vi "Get Referenced NI-XNET Port Item IDs.vi"(8 "Error In":errorcluster, 10 "CD Port Item Ref In":T1 format="%.0x", 11 "Device Item Ref in in":T1 format="%.0x") -> (0 "Error Out":errorcluster, 1 "NI-XNET Port Item Ref Out":T1 format="%.0x", 3 "Device Item Ref out":T1 format="%.0x", 4 "Found?":bool)   [LabVIEW 2017, in "NI-XNET Monitor System Explorer.lvlib"]
uses:
  NI-XNET Monitor System Explorer.lvlib
  <vilib>/NI Veristand/Custom Device API/Custom Device Item Ref.ctl
  Shared/Constants.vi
  <vilib>/NI Veristand/Custom Device API/Get Item Property (String).vi
  <vilib>/NI Veristand/Custom Device API/Custom Device API.lvlib
  Shared/NI-XNET Monitor Shared.lvlib
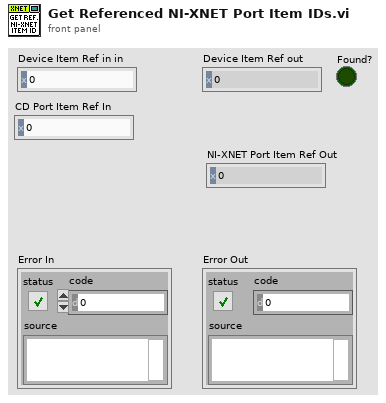
[diagram p1: front panel]
types:
  T1 = typedef "Custom Device API.lvlib/Custom Device Item Ref.ctl" = u64
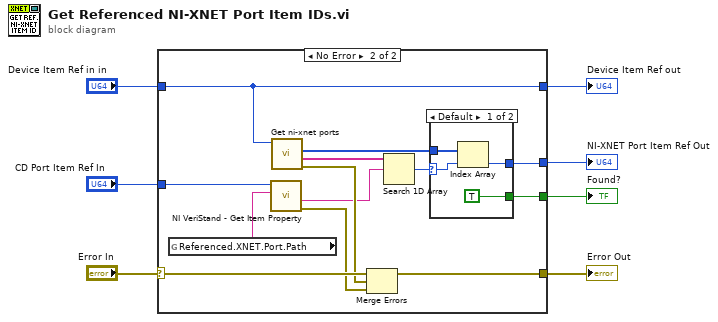
[diagram p0: block diagram]
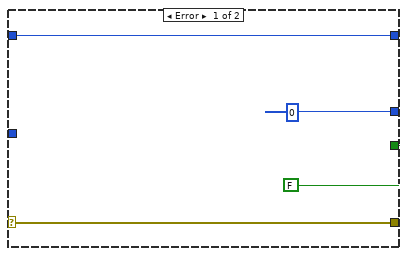
[diagram p2: hidden frame]
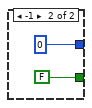
[diagram p3: hidden frame]
diagram:
  n1 = case shown="No Error" "Error In" {
    selector: "Error In" -> [w9 w24]
    tunnel: [w9 w23] -> w5
    tunnel: "Device Item Ref in in" -> [w11 w21]
    tunnel: [w11 w21] -> w7
    tunnel: "CD Port Item Ref In" -> [_ w17]
    tunnel: [T1 0 ("CD Port Item Ref In") w14] -> w2
    tunnel: [FALSE w13] -> w1
    frame Error {
    }
    frame No Error {
      n2 = global read "Constants.vi" "Referenced.XNET.Port.Path"() -> (w18:string)
      n3 = call-poly <vilib>:"NI VeriStand - Get Item Property.vi"("Property Name"=w18, "Item Ref in"=w17) -> ("error out"=w16:errorcluster, "Value"=w15:string)  [unwired: 6 in, 2 out]
      n4 = call "Get ni-xnet ports.vi"("Device Item Ref in"=w21) -> ("Error Out"=w22:errorcluster, "NI-XNET Port Item Paths"=w20:string[], "NI-XNET Port Refs"=w19:T1[])  [unwired: 7 in, 1 out]
      n5 = Merge Errors(w24, w22, w16) -> (w23:errorcluster)
      n6 = Search 1D Array(1D array=w20, element=w15) -> (index of element=w12:i32)  [unwired: 1 in]
      n7 = case shown="Default" w12 {
        selector: w12 -> [w27 _]
        tunnel: w19 -> [w28 _]
        tunnel: [w26 T1 0 ("CD Port Item Ref In")] -> w14
        tunnel: [TRUE FALSE] -> w13
        frame Default {
          n8 = Index Array(array=w28, index=w27) -> (element=w26:T1)
        }
        frame -1 {
        }
      }
    }
  }
  "Device Item Ref out" <- w7
  "Error Out" <- w5
  "NI-XNET Port Item Ref Out" <- w2
  "Found?" <- w1
